vi "SH_InfoGain.vi"(8 "error in (no error)":errorcluster, 9 "NumberOfClasses":i32, 10 "Class Labels":string[](array[string]), 11 "Distancies":dbl[][](array[numeric])) -> (0 "error out":errorcluster, 3 "Accuracy":sgl format="%.2f")   [LabVIEW 2016, in "Shapelets Search (Brute Force).lvlib"]
uses:
  <vilib>/vision/Classification.llb/IMAQ Classifier Nearest Neighbor options.ctl
  Shapelets Search (Brute Force).lvlib
  <vilib>/vision/NI_Vision_Development_Module.lvlib
panel:
  # "This VI is a part of BCI Design library, http://www.ru-bci.org \nCopyright © 2020, Sotnikov Peter, All rights reserved. License: GNU GPLv3"
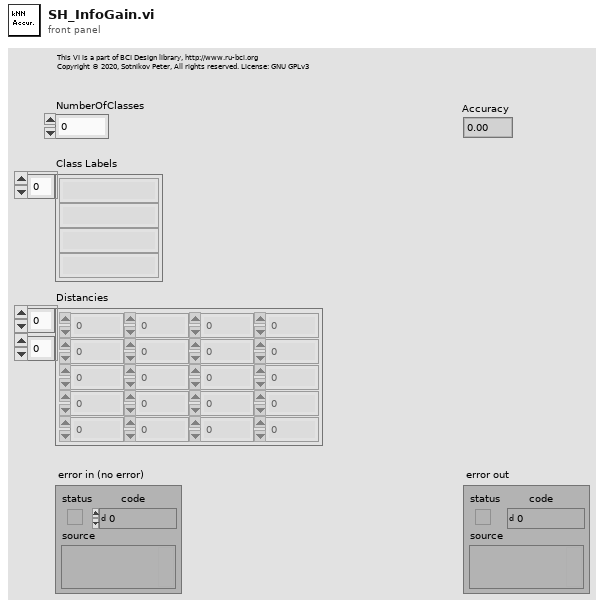
[diagram p1: front panel]
types:
  T1 = typedef "IMAQ Classifier Nearest Neighbor options.ctl" = cluster{"Method":i32, "Metric":i32, "k":i32}
  T2 = typedef "IMAQ Classifier Session.ctl" = refnum<k1>
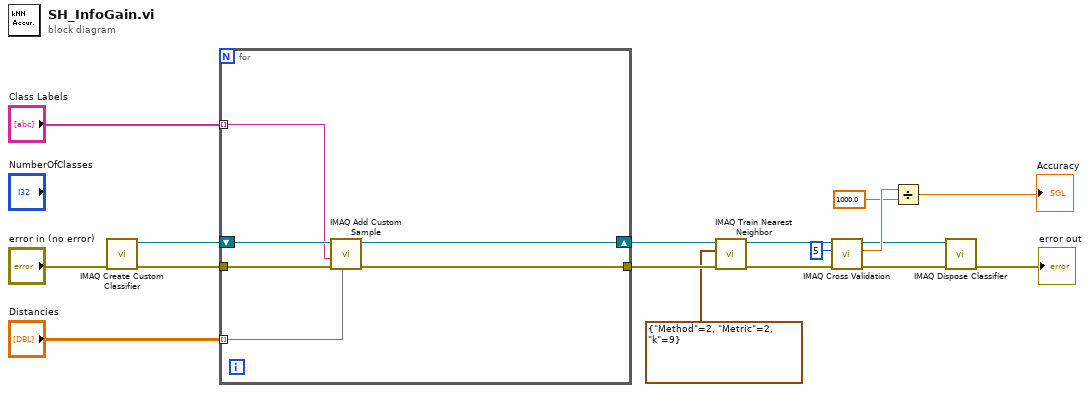
[diagram p0: block diagram]
diagram:
  n1 = call "IMAQ Create Custom Classifier"("error in (no error)"="error in (no error)") -> ("error out"=w15:errorcluster, "Classifier Session"=w17:T2)  [unwired: 9 in]
  n2 = for {
    tunnel: w15 -> [w23]
    tunnel: "Class Labels" -> [w21] mode=indexing
    tunnel: "Distancies" -> [w20] mode=indexing
    tunnel: [w18] -> w11
    shift-right: [w19] -> w12
    shift-left: w17 -> [w22]
    n3 = call "IMAQ Add Custom Sample"("Feature Vector"=w20, "error in (no error)"=w23, "Class"=w21, "Classifier Session"=w22) -> ("error out"=w18:errorcluster, "Classifier Session (dup)"=w19:T2)  [unwired: 6 in]
  }
  n4 = call "IMAQ Train Nearest Neighbor"("error in (no error)"=w11, "Nearest Neighbor Options"=T1 {"Method"=2, "Metric"=2, "k"=9}, "Classifier Session"=w12) -> ("error out"=w1:errorcluster, "Classifier Session (dup)"=w4:T2)  [unwired: 5 in, 2 out]
  n5 = call "IMAQ Cross Validation"("error in (no error)"=w1, "K - Value"=u32 5, "Classifier Session"=w4) -> ("error out"=w2:errorcluster, "Cross Validation Accuracy"=w7:dbl, "Classifier Session (dup)"=w3:T2)  [unwired: 4 in]
  n6 = Divide(x=w7, y=1000.0) -> (x/y=→"Accuracy":dbl)
  n7 = call "IMAQ Dispose Classifier"("error in (no error)"=w2, "Classifier Session"=w3) -> ("error out"=→"error out":errorcluster)  [unwired: 9 in]
